vi "PH_PILS.enable MainAmp.vi"(0 "i ref in":refnum<vi>, 5 "error in":errorcluster) -> (14 "i ref out":refnum<vi>, 19 "error out":errorcluster)   [LabVIEW 2014, in "PH_PILS.lvlib"]
uses:
  PH_PILS.lvlib
  PH_Common/PH_Common.lvlib
  PH_SystemInformation/PH_SystemInformation.lvlib
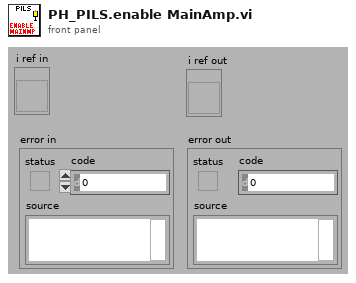
[diagram p1: front panel]
types:
  T1 = typedef "PH_PILS.lvlib/PH_PILS.i attribute.ctl" = cluster{"Boolean":cluster{"GUI Ref":refnum<vi>, "Status":i32}[], "GUI Refs Exp. Shutters":cluster{"1":refnum<vi>, "2":refnum<vi>, "3":refnum<vi>, "4":refnum<vi>}, "Tristate2Run GUI Refs":refnum<vi>[], "EO-Likes":cluster{"GUI Ref":refnum<vi>, "Status":i32}[], "Operation Mode":cluster{"Operation Mode":T2, "GUI":cluster{"Ref State":refnum<vi>, "Ref":refnum<vi>}, "Servicemode":cluster{"Tagname":string, "Status":i32}, "Labormode":cluster{"Tagname":string, "Status":i32}, "Searchmode":cluster{"Tagname":string, "Status":i32}, "Shotmode":cluster{"Tagname":string, "Status":i32}}, "Submode":cluster{"Submode":T3, "GUI":cluster{"Ref State":refnum<vi>, "Ref":refnum<vi>}, "Submode":cluster{"Tagname":string, "Status":i32}}, "Experiment":cluster{"Experiment":enum16{"unknown", "intern", "4 (Z6)", "3", "2", "1"}, "GUI":cluster{"Ref State":refnum<vi>, "Ref":refnum<vi>}, "intern":cluster{"Tagname":string, "Status":i32}, "Exp 4":cluster{"Tagname":string, "Status":i32}, "Exp 3":cluster{"Tagname":string, "Status":i32}, "Exp 2":cluster{"Tagname":string, "Status":i32}, "Exp 1":cluster{"Tagname":string, "Status":i32}}, "TristateNormal":cluster{"GUI Ref":refnum<vi>, "Status":i32}[], "Door Tags":cluster{"GUI Ref":refnum<vi>, "Status":i32}[], "GUIlessTags":cluster{"Name":string, "Status":i32}[], "Beamline GUI Refs":refnum<vi>[], "Special Boolean":cluster{"GUI Ref":refnum<vi>, "Status":i32}[], "Laserpower":cluster{"GUI Ref":refnum<vi>, "Status":i32}[], "Shutter":cluster{"GUI Ref":refnum<vi>, "Status":i32}[], "Tristate EO Like":cluster{"GUI Ref":refnum<vi>, "Status":i32}[], "PP":cluster{"GUI Ref":refnum<vi>, "Status":i32, "Head Ref":refnum<vi>, "Slider Ref":refnum<vi>}[], "Switch Knobs":cluster{"GUI Ref":refnum<vi>, "Status":i32}[], "Latch Knob GUI Refs":refnum<vi>[], "FailureCounter":i32, "Enabled Status":cluster{"Laser":i32, "PreAmp":i32, "MainAmp":i32}, "Mercury":refnum<vi>, "Instance Rods":string, "Logfile":path, "Beckhoff-Instance Internal":string, "Beckhoff-Instance External":string, "Enabling Rights":cluster{"Name":string, "Password":string, "PA?":bool, "MA?":bool, "Exp?":bool}[]}
  T2 = typedef "PH_PILS.lvlib/PH_PILS.Operation Mode.ctl" = enum16{"unknown", "Service", "Labor", "Search", "Shot"}
  T3 = typedef "PH_PILS.lvlib/PH_PILS.Submode.ctl" = enum16{"unknown", "HV-Normal", "HV-Test"}
  T4 = enum16{"Laser", "PreAmp", "MainAmp", "Exp 1", "Exp 2", "Exp 3", "Exp 4"}
  T5 = typedef "PH_SystemInformation.lvlib/PH_SystemInformationEnabling State.ctl" = i32
  T6 = typedef "PH_SystemInformation.lvlib/PH_SystemInformation.i attribute.ctl" = cluster{"Laser Enabling":cluster{"GUI Ref":refnum<vi>, "Enabling State":T5}, "PreAmp Enabling":cluster{"GUI Ref":refnum<vi>, "Enabling State":T5}, "MainAmp Enabling":cluster{"GUI Ref":refnum<vi>, "Enabling State":T5}, "Emergency Off":cluster{"GUI Ref":refnum<vi>, "State":enum16{"no info", "off/false", "Alarm"}}, "Enabling Exp. 1":cluster{"GUI Ref":refnum<vi>, "Enabling State":T5}, "Enabling Exp. 2":cluster{"GUI Ref":refnum<vi>, "Enabling State":T5}, "Enabling Exp. 3":cluster{"GUI Ref":refnum<vi>, "Enabling State":T5}, "Enabling Exp. 4":cluster{"GUI Ref":refnum<vi>, "Enabling State":T5}, "Timing Mode":cluster{"GUI Ref":refnum<vi>, "PHELIX_Timing_Mode":enum32{"10 Hz", "0.5 Hz", "Shot"}}}
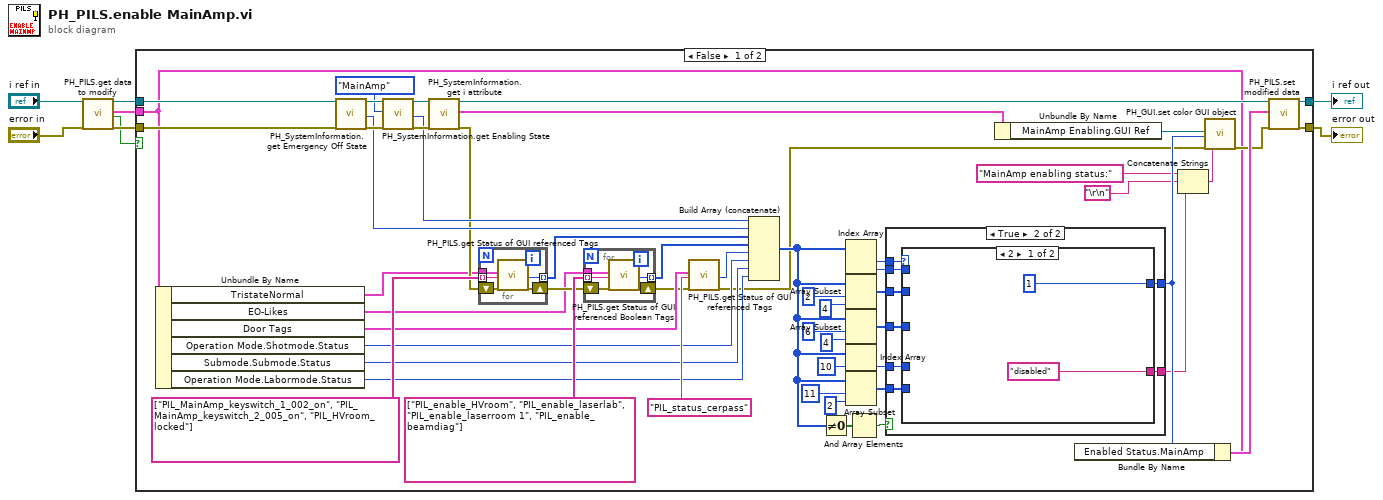
[diagram p0: block diagram]
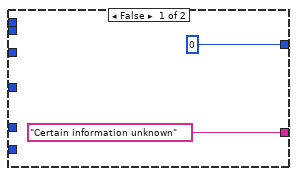
[diagram p2: hidden frame]
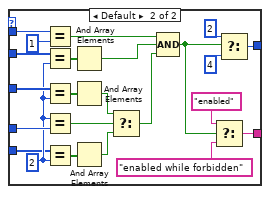
[diagram p3: hidden frame]
diagram:
  n1 = call "PH_PILS.get data to modify.vi"("i ref in"="i ref in", "error in (no error)"="error in") -> ("i ref out"=w4:refnum<vi>, "i attribute"=w5:T1, "timed out"=w3:bool, "error out"=w7:errorcluster)  [unwired: 14 in]
  n2 = case shown="False" w3 {
    tunnel: w7 -> [w19 w108]
    tunnel: w5 -> [w14 _]
    tunnel: [w60 w108] -> w2
    tunnel: w4 -> [w17 w109]
    tunnel: [w59 w109] -> w1
    frame False {
      n3 = Unbundle By Name(w14) -> ("TristateNormal"=w13:cluster{"GUI Ref":refnum<vi>, "Status":i32}[], "EO-Likes"=w15:cluster{"GUI Ref":refnum<vi>, "Status":i32}[], "Door Tags"=w42:cluster{"GUI Ref":refnum<vi>, "Status":i32}[], "Operation Mode.Shotmode.Status"=w30:i32, "Submode.Submode.Status"=w39:i32, "Operation Mode.Labormode.Status"=w38:i32)
      n4 = call "PH_SystemInformation.get Emergency Off State.vi"("i ref in"=w17, "error in (no error)"=w19) -> ("i ref out"=w28:refnum<vi>, "Emergency Off State"=w20:enum16{"no info", "off/false", "Alarm"}, "error out"=w27:errorcluster)  [unwired: 15 in]
      n5 = call "PH_SystemInformation.get Enabling State.vi"("i ref in"=w28, "Wanted State"=T4."MainAmp", "error in (no error)"=w27) -> ("i ref out"=w29:refnum<vi>, "Enabling State"=w21:T5, "error out"=w25:errorcluster)  [unwired: 14 in]
      n6 = call "PH_SystemInformation.get i attribute.vi"("i ref in"=w29, "error in (no error)"=w25) -> ("i ref out"=w16:refnum<vi>, "i attribute"=w22:T6, "error out"=w18:errorcluster)  [unwired: 15 in]
      n7 = for {
        tunnel: w13 -> [w63]
        tunnel: string[] ["PIL_MainAmp_keyswitch_1_002_on", "PIL_MainAmp_keyswitch_2_005_on", "PIL_HVroom_locked"] -> [w66] mode=indexing
        tunnel: [w67] -> w44 mode=indexing
        shift-right: [w65] -> w45
        shift-left: w18 -> [w64]
        n8 = call "PH_PILS.get Status of GUI referenced Tags.vi"("Tags"=w63, "Tagname"=w66, "error in"=w64) -> ("Status"=w67:i32, "error out"=w65:errorcluster)  [unwired: 13 in, 2 out]
      }
      n9 = for {
        tunnel: w15 -> [w68]
        tunnel: string[] ["PIL_enable_HVroom", "PIL_enable_laserlab", "PIL_enable_laserroom 1", "PIL_enable_beamdiag"] -> [w71] mode=indexing
        tunnel: [w72] -> w43 mode=indexing
        shift-right: [w70] -> w41
        shift-left: w45 -> [w69]
        n10 = call "PH_PILS.get Status of GUI referenced Boolean Tags.vi"("Tags"=w68, "Tagname"=w71, "error in"=w69) -> ("Status"=w72:i32, "error out"=w70:errorcluster)  [unwired: 13 in, 2 out]
      }
      n11 = call "PH_PILS.get Status of GUI referenced Tags.vi"("Tags"=w42, "Tagname"="PIL_status_cerpass" ("element"), "error in"=w41) -> ("Status"=w40:i32, "error out"=w23:errorcluster)  [unwired: 13 in, 2 out]
      n12 = Build Array (concatenate)(w21, w20, w44, w43, w40, w30, w39, w38) -> (w34:T5[])
      n13 = Not Equal To 0?(x=w34) -> (x != 0?=w62:bool[])
      n14 = Index Array(array=w34) -> (element #1=w53:T5, element #2=w37:T5)  [unwired: 2 in]
      n15 = Array Subset(array=w34, index=2, length=4) -> (w50:T5[])
      n16 = Array Subset(array=w34, index=6, length=4) -> (w47:T5[])
      n17 = Index Array(array=w34, index=10) -> (element=w36:T5)
      n18 = Array Subset(array=w34, index=11, length=2) -> (w31:T5[])
      n19 = And Array Elements(Boolean array=w62) -> (logical AND=w61:bool)
      n20 = case shown="True" w61 {
        tunnel: [0 ("Status") w82] -> w56
        tunnel: w53 -> [_ w78]
        tunnel: w37 -> [_ w81]
        tunnel: w50 -> [_ w80]
        tunnel: w47 -> [_ w79]
        tunnel: w36 -> [_ w77]
        tunnel: w31 -> [_ w76]
        tunnel: ["Certain information unknown" w75] -> w9
        frame False {
        }
        frame True {
          n21 = case shown="2" w78 {
            tunnel: [1 ("y") w107] -> w82
            tunnel: w81 -> [_ w105]
            tunnel: w80 -> [_ w104]
            tunnel: w79 -> [_ w103]
            tunnel: w77 -> [_ w94]
            tunnel: w76 -> [_ w92]
            tunnel: ["disabled" w88] -> w75
            frame 2 {
            }
            frame Default {
              w93 = 2 ("y")
              n22 = Equal?(x=w105, y=1) -> (x = y?=w101:bool)
              n23 = Equal?(x=w104, y=w93) -> (x = y?=w100:bool[])
              n24 = Equal?(x=w103, y=w93) -> (x = y?=w102:bool[])
              n25 = Equal?(x=w93, y=w94) -> (x = y?=w90:bool)
              n26 = Equal?(x=w92, y=w93) -> (x = y?=w91:bool[])
              n27 = And Array Elements(Boolean array=w100) -> (logical AND=w97:bool)
              n28 = And Array Elements(Boolean array=w102) -> (logical AND=w96:bool)
              n29 = And Array Elements(Boolean array=w91) -> (logical AND=w89:bool)
              n30 = Select(t=w96, s=w90, f=w89) -> (s? t:f=w95:bool)
              n31 = Compound Arithmetic op=AND(w101, w97, w95) -> (w87:bool)
              n32 = Select(t="enabled", s=w87, f="enabled while forbidden") -> (s? t:f=w88:string)
              n33 = Select(t=2 ("y"), s=w87, f=4 ("y")) -> (s? t:f=w107:i32)
            }
          }
        }
      }
      n34 = Unbundle By Name(w22) -> ("MainAmp Enabling.GUI Ref"=w24:refnum<vi>)
      n35 = Bundle By Name(cluster=w14, "Enabled Status.MainAmp"=w56) -> (w58:T1)
      n36 = Concatenate Strings("MainAmp enabling status:", "\r\n", w9) -> (w12:string)
      n37 = call "PH_GUI.set color GUI object.vi"("GUI object Ref"=w24, "State"=w56, "error in (no error)"=w23, "Tip Strip (N/A)"=w12) -> ("error out"=w57:errorcluster)  [unwired: 15 in]
      n38 = call "PH_PILS.set modified data.vi"("i ref in"=w16, "i attribute"=w58, "error in (no error)"=w57) -> ("i ref out"=w59:refnum<vi>, "error out"=w60:errorcluster)  [unwired: 15 in]
    }
    frame True {
    }
  }
  "i ref out" <- w1
  "error out" <- w2
